vi "ERD_JSON_CentUI - Add File Globals to Sequence.vi"(0 "Sequence Context In":refnum<k7>, 5 "Build":string, 7 "ERD JSON File":path, 11 "Error In":errorcluster) -> (15 "Error Out":errorcluster)   [LabVIEW 2016]
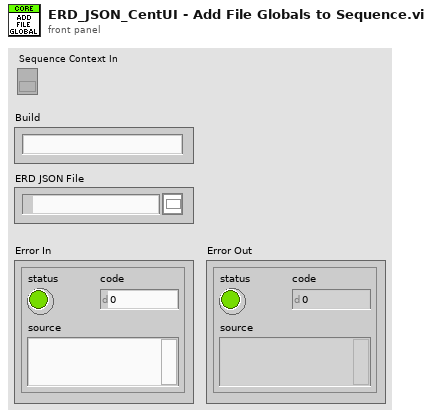
[diagram p1: front panel]
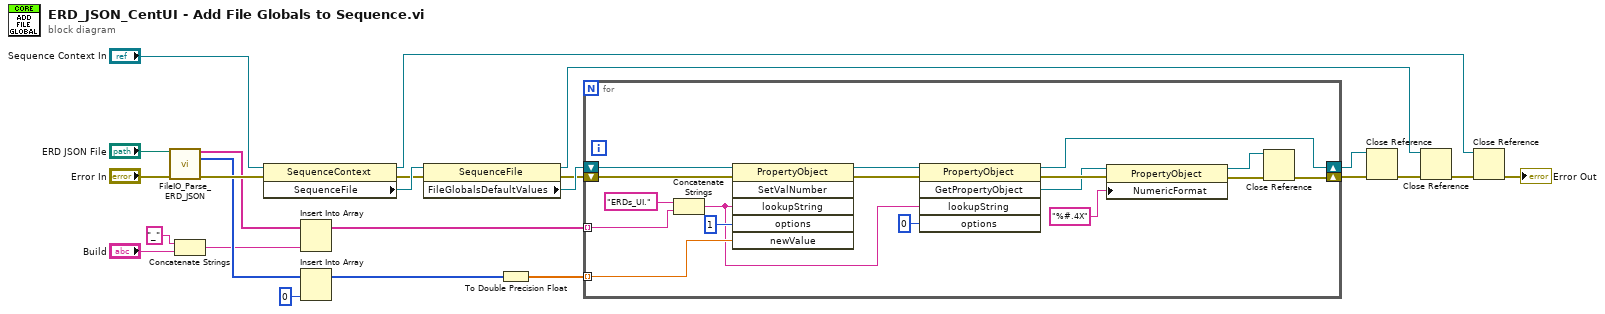
[diagram p0: block diagram]
diagram:
  n1 = call "FileIO_Parse_ERD_JSON.vi"("ERD JSON File"="ERD JSON File", "Error In"="Error In") -> ("ERD Names"=w8:string[], "ERD Numbers"=w7:u16[], "Error Out"=w13:errorcluster)  [unwired: 10 in, 1 out]
  n2 = Concatenate Strings("_" ("string"), "Build") -> (w4:string)
  n3 = property class="SequenceContext"(reference="Sequence Context In", error in=w13) -> (reference out=w14:refnum<k7>, error out=w22:errorcluster, "SequenceFile"=w23:refnum<k7>)
  n4 = Insert Into Array(array=w8, new element=w4) -> (w1:string[])  [unwired: 1 in]
  n5 = Insert Into Array(array=w7, new element=u16 0 ("new element/subarray")) -> (w2:u16[])  [unwired: 1 in]
  n6 = property class="SequenceFile"(reference=w23, error in=w22) -> (reference out=w16:refnum<k7>, error out=w20:errorcluster, "FileGlobalsDefaultValues"=w21:refnum<k7>)
  n7 = To Double Precision Float(number=w2) -> (double precision float=w10:dbl[])
  n8 = for {
    shift-right: [w27] -> w18
    shift-left: w20 -> [w39]
    shift-right: [w28] -> w19
    shift-left: w21 -> [w40]
    tunnel: w1 -> [w25] mode=indexing
    tunnel: w10 -> [w38] mode=indexing
    n9 = Concatenate Strings("ERDs_UI.", w25) -> (w34:string)
    n10 = invoke class="PropertyObject" method="SetValNumber"(reference=w40, error in=w39, "lookupString"=w34, "options"=1, "newValue"=w38) -> (reference out=w35:refnum<k7>, error out=w36:errorcluster)  [unwired: 1 in, 4 out]
    n11 = invoke class="PropertyObject" method="GetPropertyObject"(reference=w35, error in=w36, "lookupString"=w34, "options"=0) -> (reference out=w28:refnum<k7>, error out=w32:errorcluster, "GetPropertyObject"=w31:refnum<k7>)  [unwired: 1 in, 2 out]
    n12 = property class="PropertyObject"(reference=w31, error in=w32, "NumericFormat"="%#.4X") -> (reference out=w29:refnum<k7>, error out=w30:errorcluster)
    n13 = Close Reference(reference=w29, error in (no error)=w30) -> (error out=w27:errorcluster)
  }
  n14 = Close Reference(reference=w19, error in (no error)=w18) -> (error out=w17:errorcluster)
  n15 = Close Reference(reference=w16, error in (no error)=w17) -> (error out=w15:errorcluster)
  n16 = Close Reference(reference=w14, error in (no error)=w15) -> (error out=→"Error Out":errorcluster)
